vi "Read TestConfiguration.vi"(8 "error in (no error)":errorcluster, 11 "TestConfiguration in":refnum<class "TestConfiguration.lvclass">) -> (0 "error out":errorcluster, 2 "TestLimit":string[][](array[string]), 3 "TestConfiguration out":refnum<class "TestConfiguration.lvclass">)   [LabVIEW 2019, in "TestSetup.lvlib" / "TestConfiguration.lvclass"]
uses:
  TestConfiguration.lvclass
  TestConfiguration.lvclass/TestConfiguration.ctl
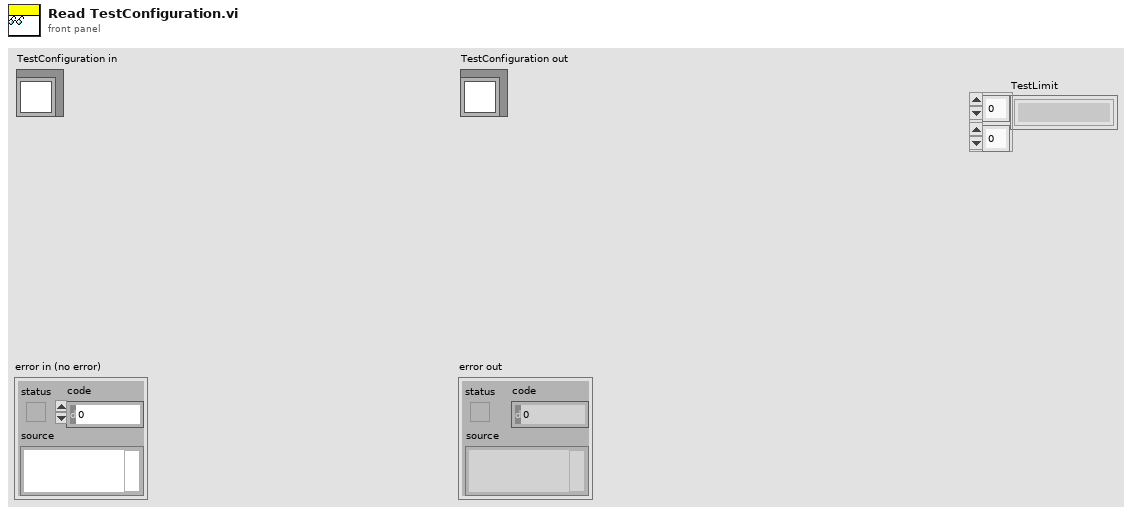
[diagram p1: front panel]
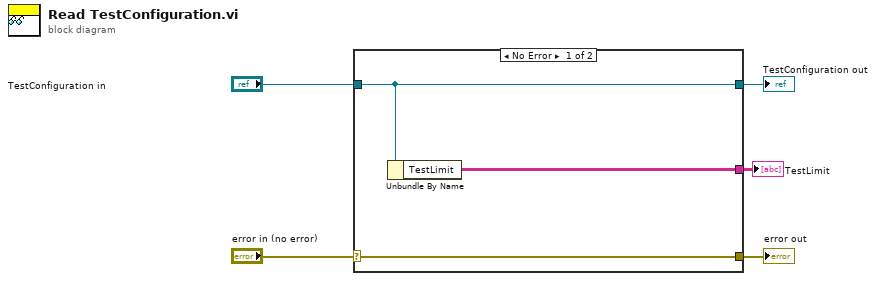
[diagram p0: block diagram]
diagram:
  n1 = case shown="No Error" "error in (no error)" {
    selector: "error in (no error)" -> [w8 w9]
    tunnel: [w8 w9] -> w4
    tunnel: [w7 w10] -> w2
    tunnel: "TestConfiguration in" -> [w7 w10]
    tunnel: [w6 _] -> w1
    frame No Error {
      n2 = Unbundle By Name(w7) -> ("TestLimit"=w6:string[][])
    }
    frame Error {
    }
  }
  "error out" <- w4
  "TestConfiguration out" <- w2
  "TestLimit" <- w1
